vi "Config Scan Variables Total.vi"(8 "error in":errorcluster, 10 "Total (0)":i32 min=0 max=99999999, 11 "VISA resource name":refnum<visa-resource-name>) -> (0 "error out":errorcluster, 3 "VISA resource name out":refnum<visa-resource-name>)   [LabVIEW 2019, in "Andeen-Hagerling 2700(400 firmware).lvlib"]
doc: "Specifies the total number of measurements to be taken when the SCAN ON command is executed. This can represent a total measurement count or the number of times that a particular scan loop is to be executed, depending on the value of the STMode parameter."
uses:
  Andeen-Hagerling 2700(400 firmware).lvlib
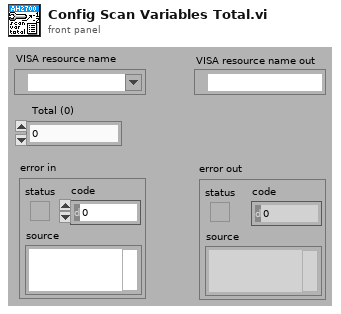
[diagram p1: front panel]
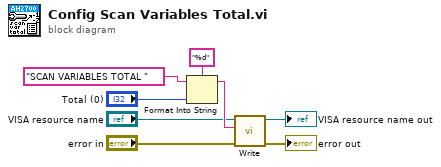
[diagram p0: block diagram]
diagram:
  n1 = Format Into String(format string="%d", initial string="SCAN VARIABLES TOTAL " ("format string"), "Total (0)") -> (resulting string=w6:string)  [unwired: 1 in, 1 out]
  n2 = call "Write.vi"("error in"="error in", "command"=w6, "VISA resource name"="VISA resource name") -> ("error out"=→"error out":errorcluster, "VISA resource name out"=→"VISA resource name out":refnum<visa-resource-name>)  [unwired: 7 in]
